vi "Read Configuration.vi"(0 "Config File Path":path, 11 "error in":errorcluster) -> (4 "Path Groups out":refnum<class "Path Group.lvclass">[](array[class]), 6 "Path Count":i32, 15 "error out":errorcluster)   [LabVIEW 2023, in "RFFixtureCharact.Public.lvlib"]
uses:
  RFFixtureCharact.Public.lvlib
  Common/Base Classes/Path Group/Path Group.lvclass
  Common/RFCalAndFixtureCharact.Common.lvlib
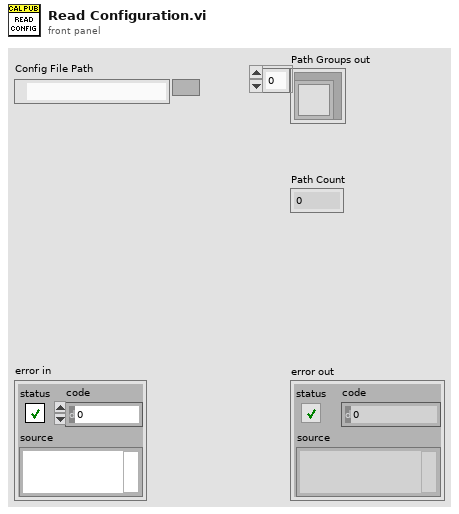
[diagram p1: front panel]
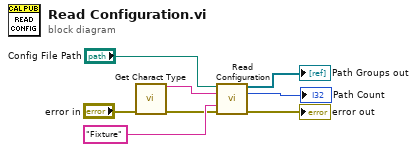
[diagram p0: block diagram]
diagram:
  n1 = call "Get Charact Type.vi"("error in (no error)"="error in") -> ("Charact type"=w1:string, "error out"=w2:errorcluster)  [unwired: 13 in]
  n2 = call "Read Configuration.vi"("Config File Path"="Config File Path", "Scalar Or Vector"=w1, "Fixture Or Cal"="Fixture", "Error in (no error)"=w2) -> ("Path Groups out"=→"Path Groups out":refnum<class "Path Group.lvclass">[], "Path Count"=→"Path Count":i32, "Error out"=→"error out":errorcluster)  [unwired: 9 in]
